vi "userauth_publickey_sign.vi"(8 "error in (no error)":errorcluster, 10 "data":u8[](array[numeric])) -> (0 "error out":errorcluster, 2 "signature":u8[](array[numeric]))   [LabVIEW 2013]
doc: "Called when authenticating with libssh2 using <B>libssh2_userauth_publickey</B>.\n\n<B>data</B> data received from the remote server.\n<B>signature</B> signature for the data to authenticated on the server."
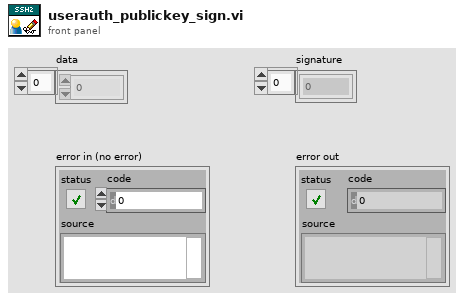
[diagram p1: front panel]
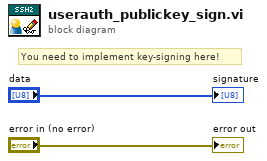
[diagram p0: block diagram]
diagram:
  # "You need to implement key-signing here!"
  "error out" <- "error in (no error)"
  "signature" <- "data"
